vi "Program LabVIEW Sistem monitoring daya V1.vi"() -> ()   [LabVIEW 2017]
uses:
  <vilib>/Instr/_visa.llb/VISA Configure Serial Port (Instr).vi
panel:
  in  "stop":bool
  out "Daya R":dbl
  out "Total Daya":dbl format="%#.0f"
  out "Total Arus":dbl(knob) scale=0.0..50.0 scale format="%#.0f"
  out "Daya T":dbl format="%#.0f"
  out "Daya S":dbl
  out "Arus T":dbl(knob) scale=0.0..10.0 scale format="%#.0f"
  out "Arus S":dbl(knob) scale=0.0..10.0 scale format="%#.0f"
  out "Arus R":dbl(knob) scale=0.0..20.0 scale format="%#.0f"
  out "Grafik Daya":cluster{dbl, dbl, dbl, dbl}(graph)
  in  "Tabel Daya (Watt)":string[][](table)
  in  "USB Port":refnum<visa-resource-name>
  # "Ampere"
  # "Ampere"
  # "Ampere"
  # "Ampere"
  # "Watt"
  # "Watt"
  # "Watt"
  # "Watt"
  # "Watt"
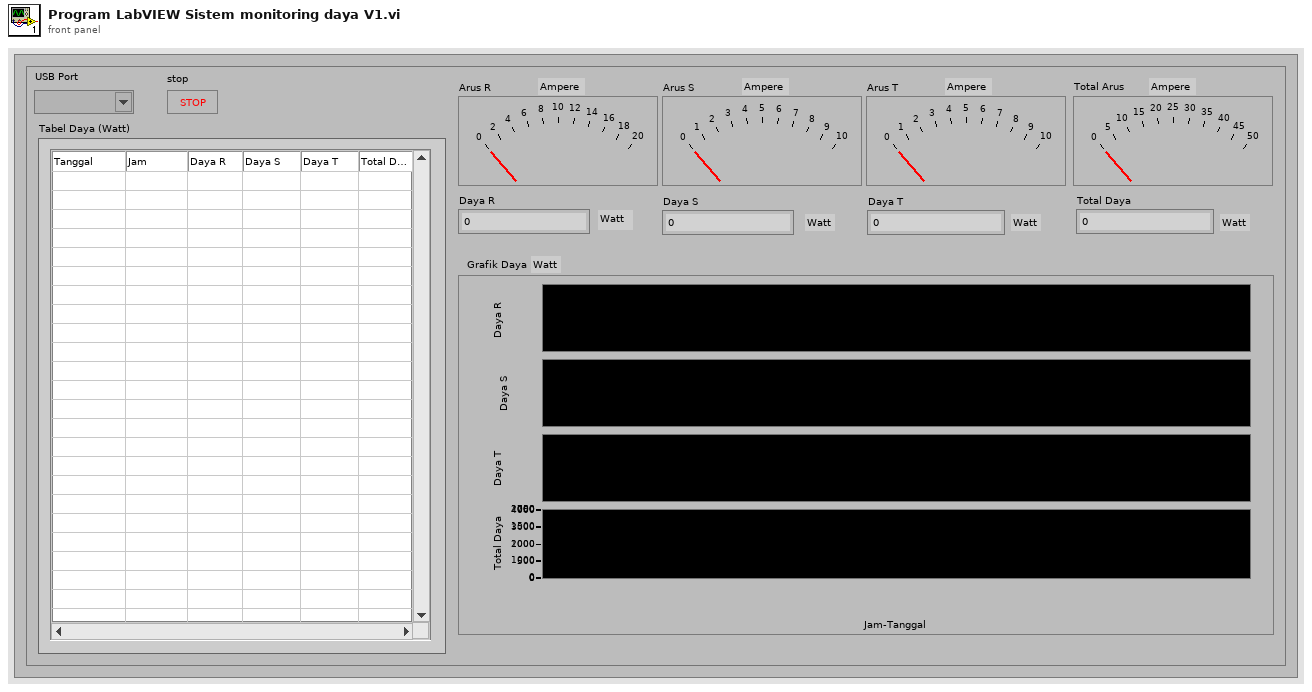
[diagram p1: front panel]
types:
  T1 = cluster{"String":dbl, "String":dbl, "String":dbl, dbl}
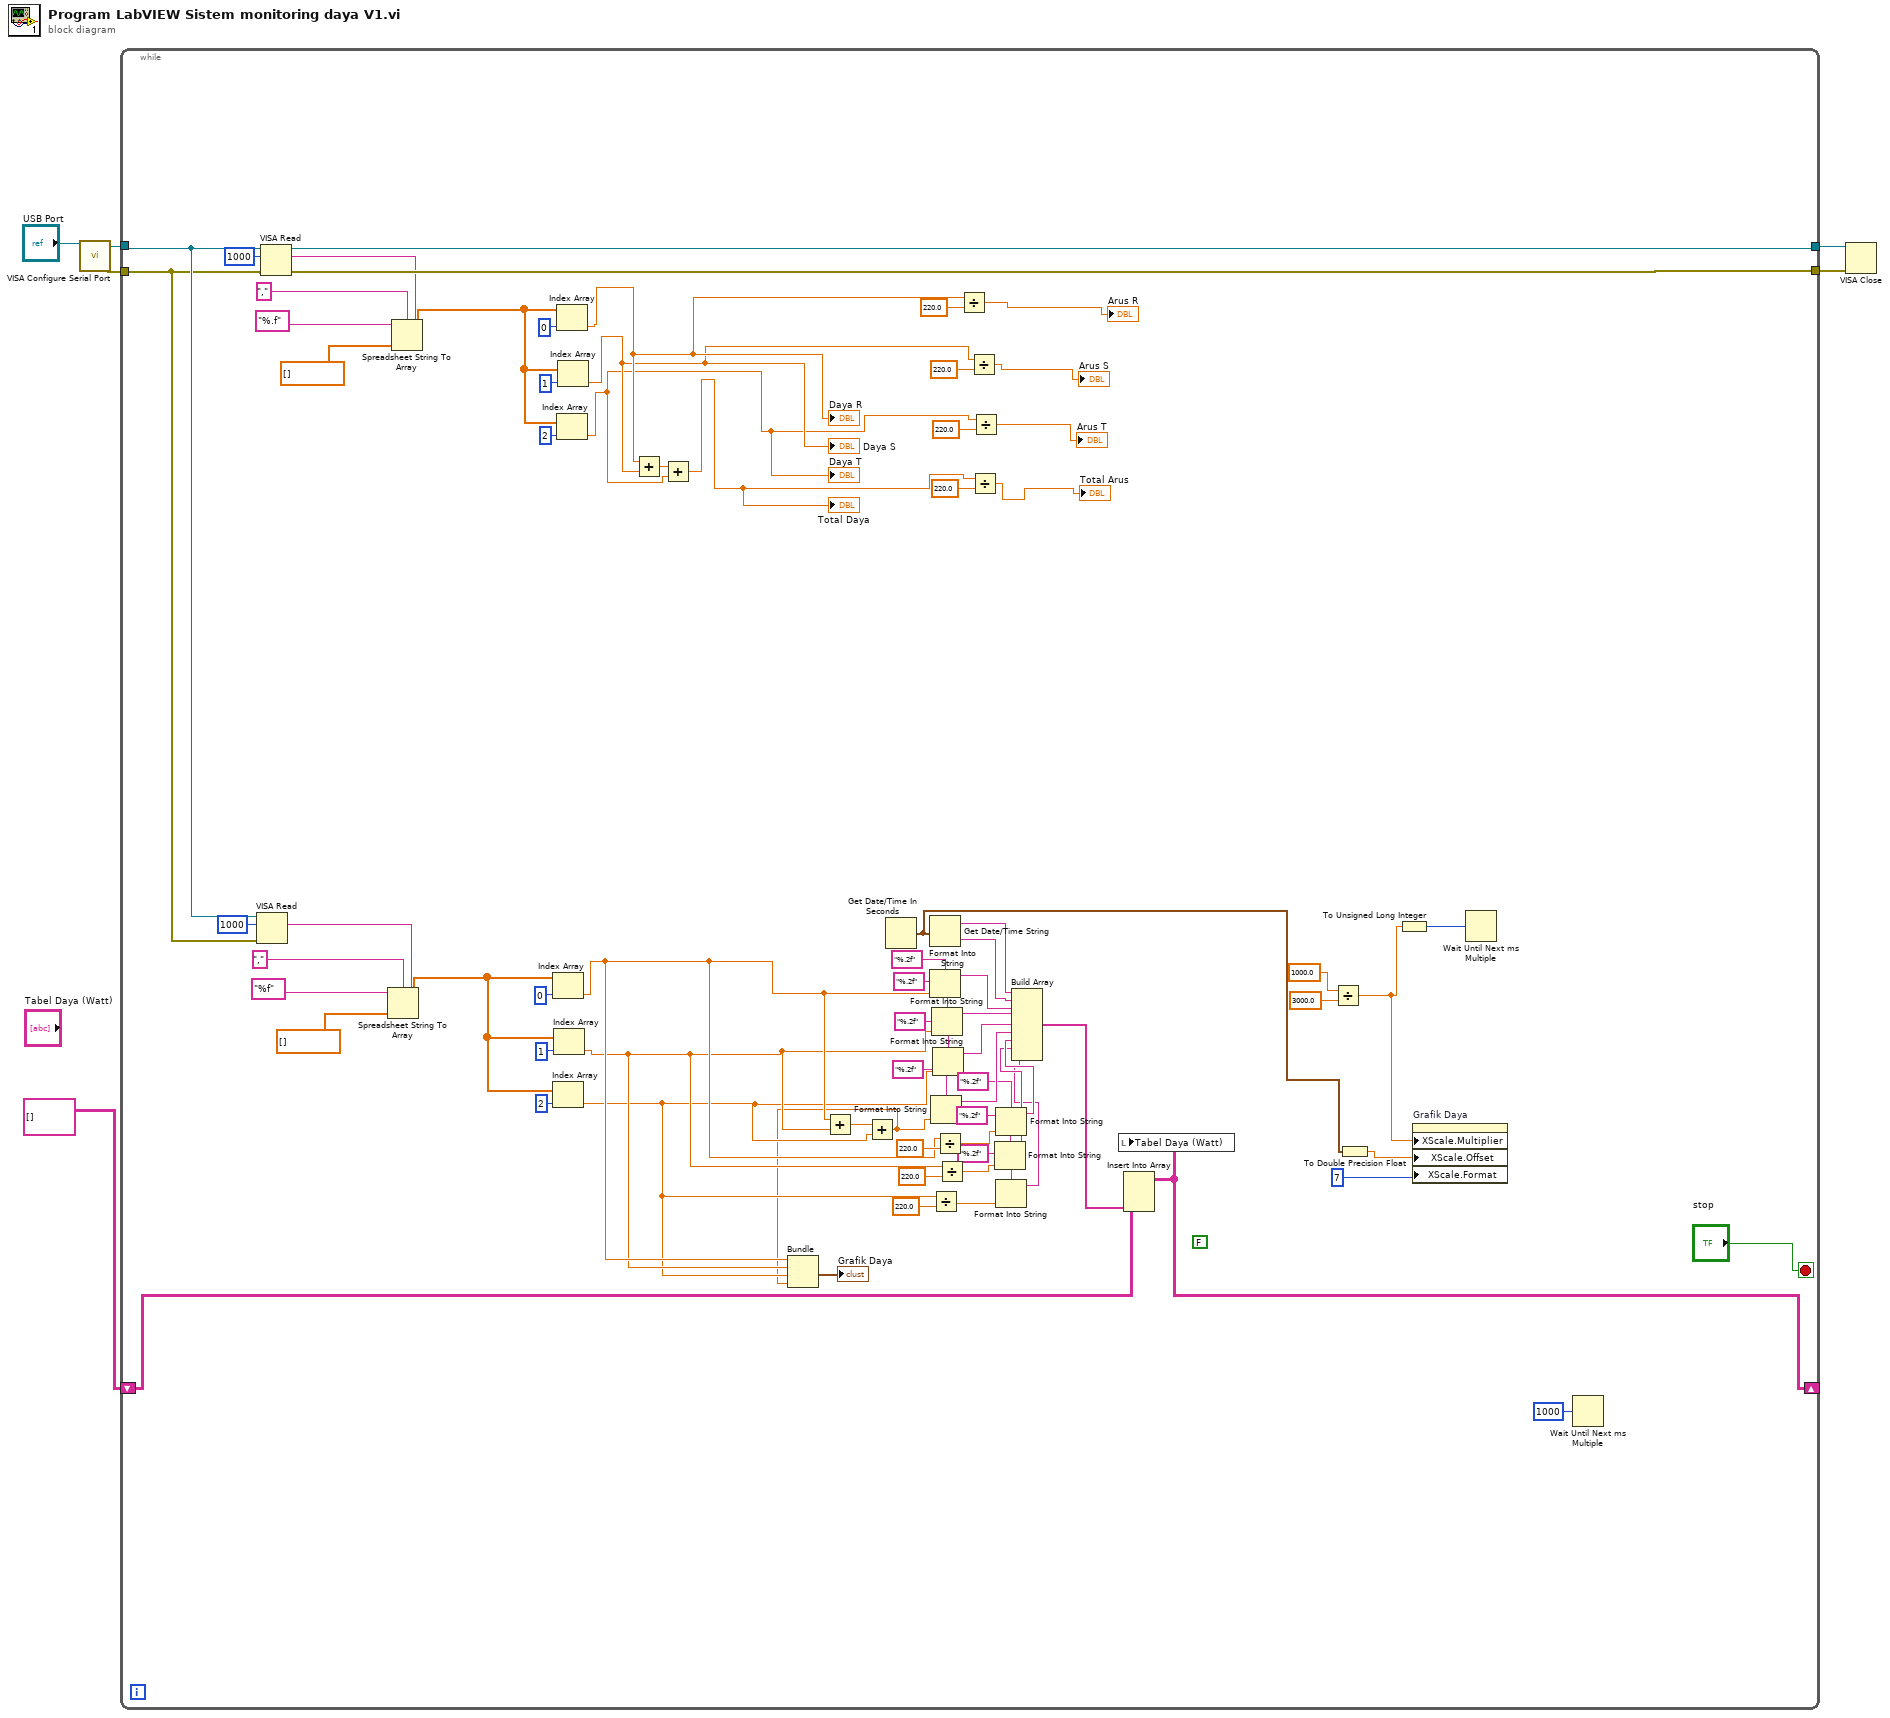
[diagram p0: block diagram]
diagram:
  n1 = call-poly "VISA Configure Serial Port"("VISA resource name"="USB Port") -> ("VISA resource name out"=w3:refnum<visa-resource-name>, "error out"=w2:errorcluster)  [unwired: 13 in]
  n2 = while {
    tunnel: [w81] -> w6
    tunnel: [w80] -> w5
    tunnel: w3 -> [w79]
    tunnel: w2 -> [w78]
    shift-right: [w30] -> _
    shift-left: string[][] [] -> [w31]
    stop <- "stop" stop-if-true
    (unwired) FALSE
    n3 = VISA Read(VISA resource name=w79, byte count=u32 1000, error in (no error)=w78) -> (read buffer=w71:string)  [unwired: 3 out]
    n4 = VISA Read(VISA resource name=w79, byte count=u32 1000, error in (no error)=w78) -> (VISA resource name out=w81:refnum<visa-resource-name>, read buffer=w23:string, error out=w80:errorcluster)  [unwired: 1 out]
    n5 = Spreadsheet String To Array(delimiter (Tab)=",", format string="%f", spreadsheet string=w71, array type (2D Dbl)=dbl[] [] ("Data Graph")) -> (array=w57:dbl[])
    n6 = Spreadsheet String To Array(delimiter (Tab)=",", format string="%.f", spreadsheet string=w23, array type (2D Dbl)=dbl[] [] ("Data Graph")) -> (array=w9:dbl[])
    n7 = Index Array(array=w57, index=0 ("disabled index (col)")) -> (element=w36:dbl)
    n8 = Index Array(array=w57, index=2 ("disabled index (col)")) -> (element=w34:dbl)
    n9 = Index Array(array=w57, index=1 ("disabled index (col)")) -> (element=w35:dbl)
    n10 = Index Array(array=w9, index=0 ("disabled index (col)")) -> (element=w20:dbl)
    "Daya R" <- w20
    n11 = Index Array(array=w9, index=2 ("disabled index (col)")) -> (element=w14:dbl)
    "Daya T" <- w14
    n12 = Index Array(array=w9, index=1 ("disabled index (col)")) -> (element=w15:dbl)
    "Daya S" <- w15
    n13 = Add(x=w20, y=w15) -> (x+y=w21:dbl)
    n14 = Add(x=w21, y=w14) -> (x+y=w8:dbl)
    "Total Daya" <- w8
    n15 = Add(x=w36, y=w35) -> (x+y=w63:dbl)
    n16 = Add(x=w63, y=w34) -> (x+y=w33:dbl)
    n17 = Bundle("String"=w36, "String"=w35, "String"=w34, w33) -> (→"Grafik Daya":T1)  [unwired: 1 in]
    n18 = Get Date/Time In Seconds() -> (seconds since 1Jan1904=w38:timestamp)
    n19 = Get Date/Time String(seconds (now)=w38) -> (date string=w65:string, time string=w64:string)  [unwired: 2 in]
    n20 = Format Into String(format string="%.2f", w36) -> (resulting string=w66:string)  [unwired: 2 in, 1 out]
    n21 = Format Into String(format string="%.2f", w33) -> (resulting string=w62:string)  [unwired: 2 in, 1 out]
    n22 = Divide(x=w34, y=220.0) -> (x/y=w51:dbl)
    n23 = Format Into String(format string="%.2f", w35) -> (resulting string=w67:string)  [unwired: 2 in, 1 out]
    n24 = Format Into String(format string="%.2f", w34) -> (resulting string=w68:string)  [unwired: 2 in, 1 out]
    n25 = Divide(x=w36, y=220.0) -> (x/y=w53:dbl)
    n26 = Divide(x=w35, y=220.0) -> (x/y=w52:dbl)
    n27 = Divide(x=w20, y=220.0) -> (x/y=→"Arus R":dbl)
    n28 = Divide(x=w15, y=220.0) -> (x/y=→"Arus S":dbl)
    n29 = Divide(x=w8, y=220.0) -> (x/y=→"Total Arus":dbl)
    n30 = Divide(x=w14, y=220.0) -> (x/y=→"Arus T":dbl)
    n31 = Format Into String(format string="%.2f", w52) -> (resulting string=w55:string)  [unwired: 2 in, 1 out]
    n32 = Format Into String(format string="%.2f", w53) -> (resulting string=w56:string)  [unwired: 2 in, 1 out]
    n33 = Format Into String(format string="%.2f", w51) -> (resulting string=w54:string)  [unwired: 2 in, 1 out]
    n34 = Build Array(w65, w64, w66, w67, w68, w62, w56, w55, w54) -> (w69:string[])
    n35 = Insert Into Array(array=w31, new element=w69) -> (w30:string[][])  [unwired: 2 in]
    n36 = local write "Tabel Daya (Watt)"(w30) -> ()
    n37 = Divide(x=1000.0, y=3000.0) -> (x/y=w43:dbl)
    n38 = To Double Precision Float(number=w38) -> (double precision float=w44:dbl)
    n39 = To Unsigned Long Integer(number=w43) -> (unsigned 32bit integer=w42:u32)
    n40 = property on="Grafik Daya" class="WFChart (strict)"("XScale.Multiplier"=w43, "XScale.Offset"=w44, "XScale.Format"=u8 7 ("X Scale.Display Format:Format")) -> ()  [unwired: 2 in, 2 out]
    n41 = Wait Until Next ms Multiple(millisecond multiple=w42) -> ()  [unwired: 1 out]
    n42 = Wait Until Next ms Multiple(millisecond multiple=u32 1000) -> ()  [unwired: 1 out]
  }
  n43 = VISA Close(VISA resource name=w6, error in (no error)=w5) -> ()  [unwired: 1 out]
